vi "ExcelDialog.vi"(8 "Labels":string[](array[string]), 9 "Center of Masses":dbl[][](array[numeric]), 11 "Band Average":dbl[][](array[numeric])) -> ()   [LabVIEW 2022 SP3]
uses:
  <vilib>/Utility/file.llb/Write Delimited Spreadsheet (string).vi
panel:
  in  "Precision":u8=2
  in  "Format":u16(ring) items=["General", "Scientific Notation"]
  in  "Save Button":bool
  in  "Close Button":bool
  out "Data Table":string[][](table)
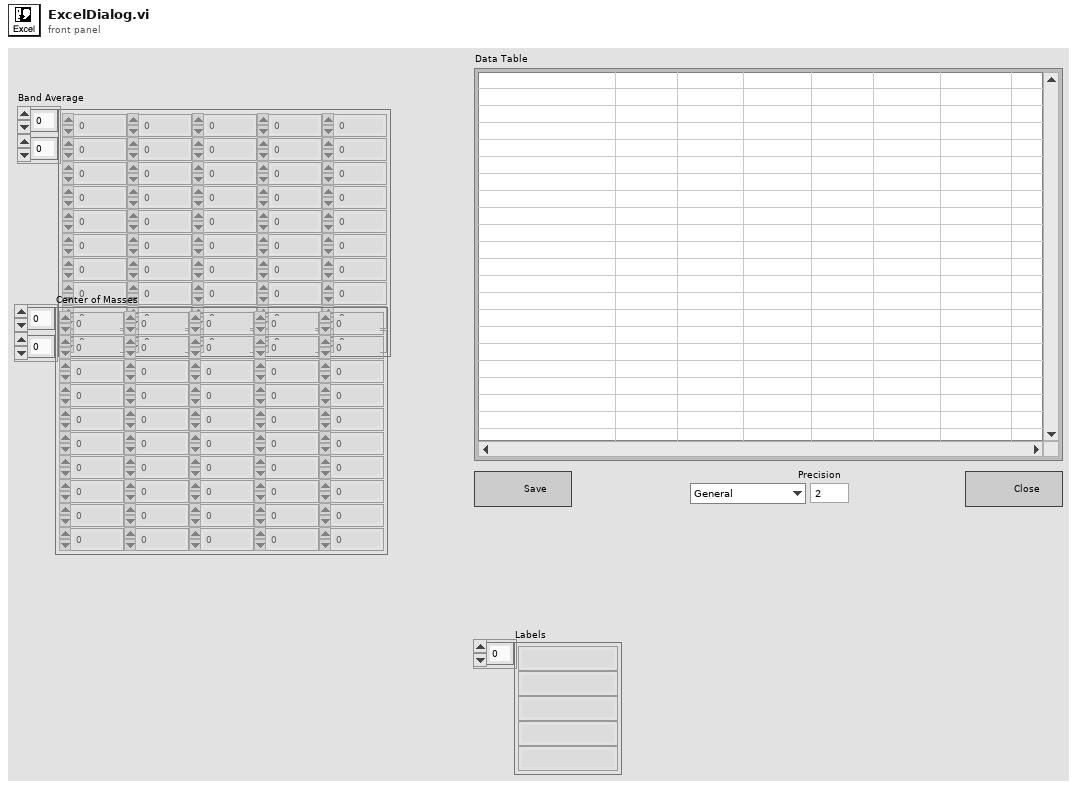
[diagram p1: front panel]
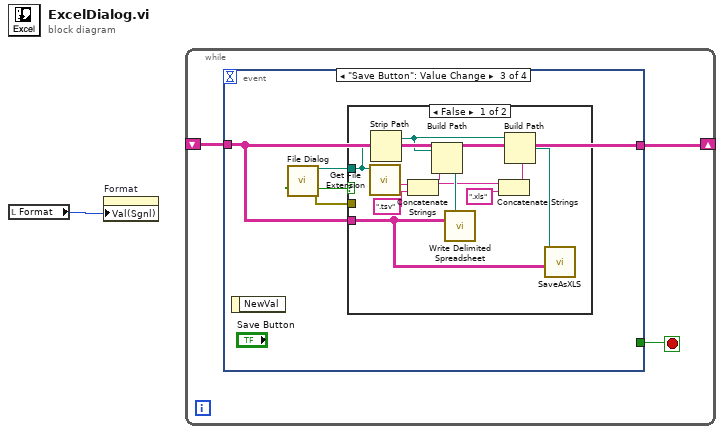
[diagram p0: block diagram]
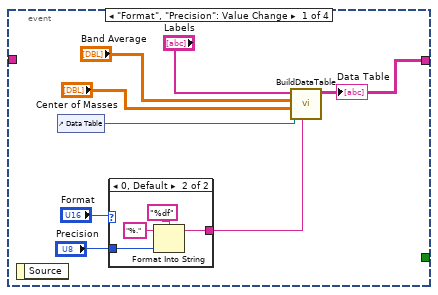
[diagram p2: hidden frame]
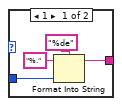
[diagram p3: hidden frame]
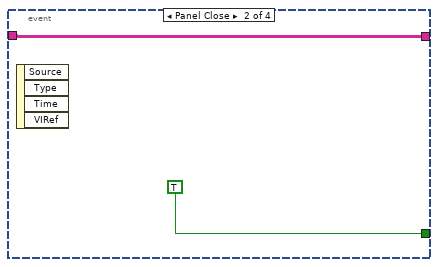
[diagram p4: hidden frame]
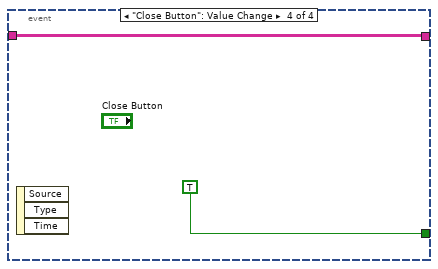
[diagram p6: hidden frame]
diagram:
  n1 = local read "Format"() -> (w1:u16)
  n2 = property on="Format" class="Ring (strict)"("Val(Sgnl)"=w1) -> ()  [unwired: 2 in, 2 out]
  n3 = while {
    shift-right: [w3] -> _
    shift-left: _ -> [w2]
    stop <- w4 stop-if-true
    n4 = event shown="[2] \"Save Button\": Value Change" {
      selector: _ -> [_ _ _ _]
      dyn-events: _ -> [_ _ _ _]
      timeout: _ -> [_ _ _ _]
      tunnel: [_ TRUE _ TRUE] -> w4
      tunnel: [w9 w21 w23 w37] -> w3
      tunnel: w2 -> [_ w21 w23 w37]
      event "Format", "Precision": Value Change {
        n5 = event-data() -> ()  [unwired: 1 in, 1 out]
        n6 = control-ref of="Data Table"() -> (w8:refnum<vi>)
        n7 = case shown="0, Default" "Format" {
          tunnel: "Precision" -> [w16 w20]
          tunnel: [w13 w17] -> w5
          frame 1 {
            n8 = Format Into String(format string="%de", initial string="%.", w16) -> (resulting string=w13:string)  [unwired: 1 in, 1 out]
          }
          frame 0, Default {
            n9 = Format Into String(format string="%df", initial string="%.", w20) -> (resulting string=w17:string)  [unwired: 1 in, 1 out]
          }
        }
        n10 = call "BuildDataTable.vi"("format string"=w5, "Table in"=w8, "Center of Masses"="Center of Masses", "Band Average"="Band Average", "Labels"="Labels") -> ("Data Table"=w9:string[][])  [unwired: 6 in]
        "Data Table" <- w9
      }
      event Panel Close {
        n11 = event-data() -> ()  [unwired: 1 in, 4 out]
      }
      event "Save Button": Value Change {
        n12 = event-data() -> ()  [unwired: 1 in, 1 out]
        n13 = call "File Dialog"() -> ("selected path"=w25:path, "cancelled"=w26:bool, "error out"=w24:errorcluster)  [unwired: 12 in, 1 out]
        n14 = case shown="False" w26 {
          tunnel: w25 -> [w35 _]
          tunnel: w23 -> [w32 _]
          tunnel: w24 -> [_ _]
          frame False {
            n15 = call <vilib>:"Get File Extension.vi"("file"=w35) -> ("filename without extension"=w30:string)  [unwired: 6 in, 4 out]
            n16 = Strip Path(path=w35) -> (stripped path=w31:path)  [unwired: 1 out]
            n17 = Concatenate Strings(w30, ".tsv" ("string")) -> (w34:string)
            n18 = Build Path(base path=w31, name or relative path=w34) -> (appended path=w33:path)
            n19 = call-poly <vilib>:"Write Delimited Spreadsheet.vi"("file path (dialog if empty)"=w33, "2D data"=w32) -> ()  [unwired: 12 in, 2 out]
            n20 = Concatenate Strings(w30, ".xls" ("string")) -> (w28:string)
            n21 = Build Path(base path=w31, name or relative path=w28) -> (appended path=w27:path)
            n22 = call "SaveAsXLS.vi"("Data Table"=w32, "file"=w27) -> ()  [unwired: 10 in]
          }
          frame True {
          }
        }
      }
      event "Close Button": Value Change {
        n23 = event-data() -> ()  [unwired: 1 in, 3 out]
      }
    }
  }
